vi "TestGenTabNameHeaders.vi"() -> ()   [LabVIEW 2014, in "TableLogger_Actor.lvlib" / "TableLogger_Actor.lvclass"]
uses:
  TableLogger_Actor.lvclass
  <userlib>/_OpenG.lib/lvdata/lvdata.llb/Type Descriptor Enumeration__ogtk.ctl
panel:
  out "LV Data Types 3":T1[](array[typedef]) format="%.0x"
  out "Headers 2":string[](array[string])
  out "Data 2":string[](array[string])
  out "LV Data Types 2":T1[](array[typedef]) format="%.0x"
  out "Table Name":string
  out "Headers":string[](array[string])
  out "Data":string[][](array[string])
  out "LV Data Types":T1[][](array[typedef]) format="%.0x"
  out "Table Names":string[](array[string])
  out "Column Headers":string[][](array[string])
  out "Column Data Types":string[][](array[string])
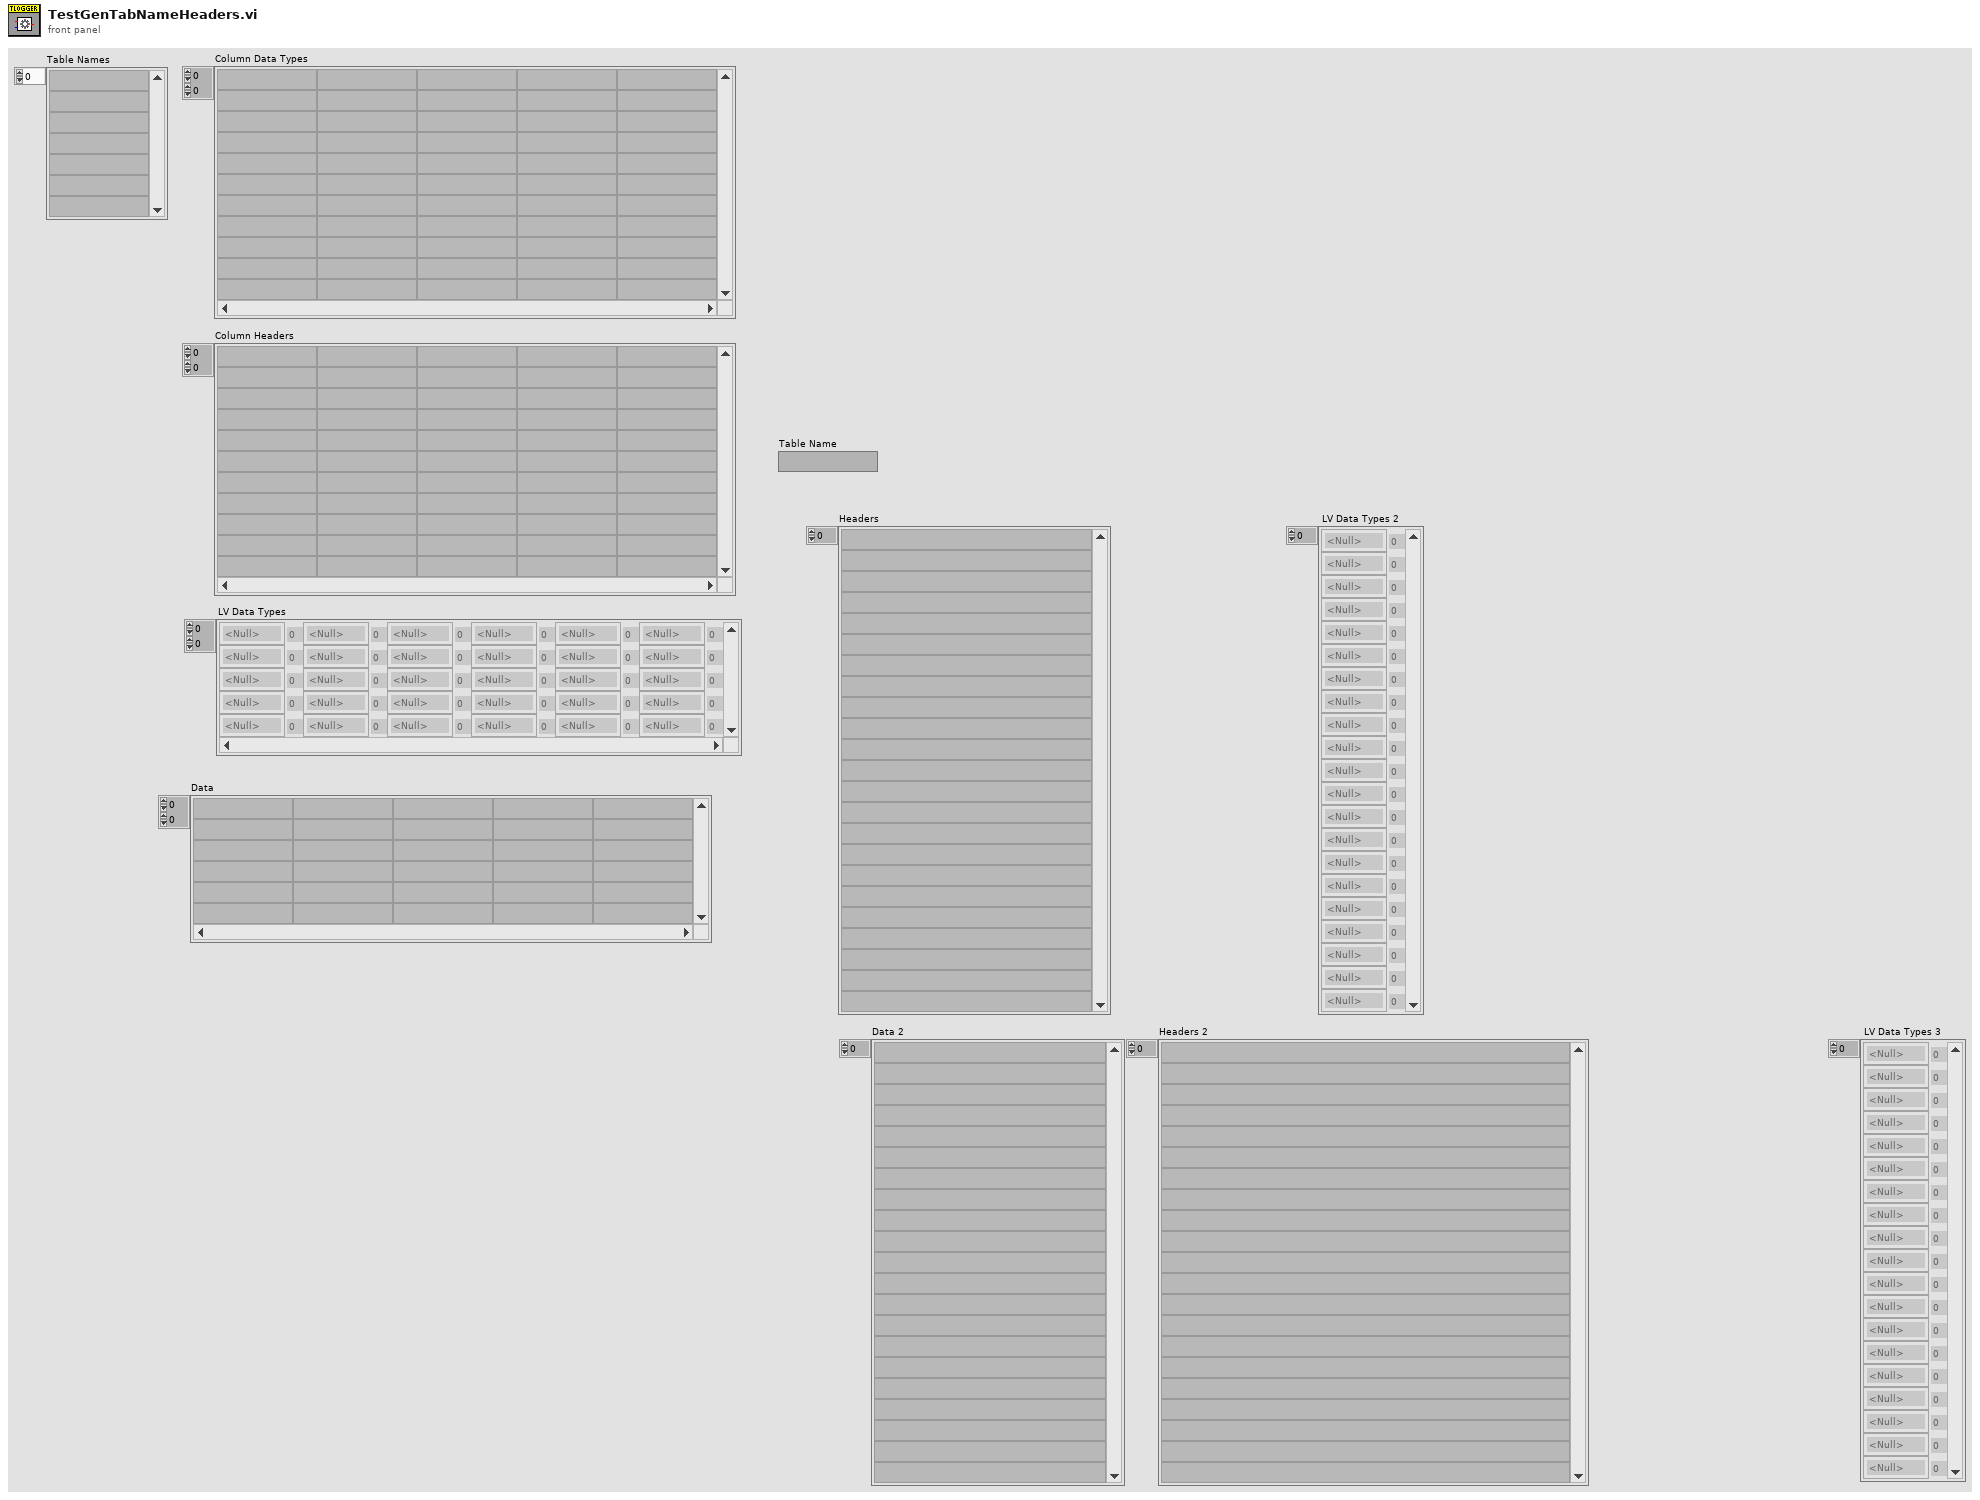
[diagram p1: front panel]
types:
  T1 = typedef "Type Descriptor Enumeration__ogtk.ctl" = enum8{"<Null>", "I8", "I16", "I32", "I64", "U8", "U16", "U32", "U64", "SGL", "DBL", "EXT", "CSG", "CDB", "CXT", "0x0F", "0x10", "0x11", "0x12", "0x13", "0x14", "Enum U8", "Enum U16", "Enum U32", "Enum U64", "SGL PQ", "DBL PQ", "EXT PQ", "CSG PQ", "CDB PQ", "CXT PQ", "0x1F", "0x20", "Boolean", "0x22", "0x23", "0x24", "0x25", "0x26", "0x27", "0x28", "0x29", "0x2A", "0x2B", "0x2C", "0x2D", "0x2E", "0x2F", "String", "0x31", "Path", "Pict", "0x34", "0x35", "0x36", "DAQ", "0x38", "0x39", "0x3A", "0x3B", "0x3C", "0x3D", "0x3E", "0x3F", "Array", "0x41", "0x42", "0x43", "0x44", "0x45", "0x46", "0x47", "0x48", "0x49", "0x4A", "0x4B", "0x4C", "0x4D", "0x4E", "0x4F", "Cluster", "0x51", "0x52", "Variant", "Waveform", "0x55", "0x56", "0x57", "0x58", "0x59", "0x5A", "0x5B", "0x5C", "0x5D", "0x5E", "0x5F", "0x60", "0x61", "0x62", "0x63", "0x64", "0x65", "0x66", "0x67", "0x68", "0x69", "0x6A", "0x6B", "0x6C", "0x6D", "0x6E", "0x6F", "Refnum"}
  T2 = cluster{"FC Flow Set":dbl, "FM Flow Measure":dbl, "UUT Data":dbl, "Stage 1  Flow Meas":cluster{"FC Flow Set":dbl, "FM Flow Measure":dbl, "UUT Data":dbl, "Dataset":cluster{"Site Number":i32, "Operator ID":string, "Calibration Result":enum16{"Pass", "Fail"}, "Stage 1  Flow Meas":cluster{"FC Flow Set":dbl, "FM Flow Measure":dbl, "UUT Data":dbl}[]}}[]}[]
  T3 = cluster{"Test Start Timestamp":timestamp, "Test End Timestamp":timestamp, "Test Jig Location":string, "Location Time Offset":string, "Test Jig ID":string, "Test Jig Fluid":enum16{"DI", "N2"}, "Test Jig Flow":enum16{"Low", "High"}, "Control Board SN":string, "Site Number":i32, "Operator ID":string, "Operation Number":string, "DUT Serial Number":string, "DUT Product Number":string, "DUT Flow Range":i32, "DUT FW Revision":string, "DUT TP1 Offset":dbl, "DUT TP2 Offset":dbl, "DUT Cut Off1":dbl, "DUT Cut Off2":dbl, "PreCal Flow Meas":cluster{"FC Flow Set":dbl, "FM Flow Measure":dbl, "UUT Data":dbl}[], "PostCal Flow Meas":cluster{"FC Flow Set":dbl, "FM Flow Measure":dbl, "UUT Data":dbl}[], "DUT_Coeff":dbl[], "DUT_Flow_Error":dbl[], "Calibration Result":enum16{"Pass", "Fail"}}
  T4 = cluster{"FC Flow Set":dbl, "FM Flow Measure":dbl, "UUT Data":dbl, "Stage 1  Flow Meas":cluster{"FC Flow Set":dbl, "FM Flow Measure":dbl, "UUT Data":dbl}[]}[]
  T5 = cluster{"Site Number":i32, "Operator ID":string, "Calibration Result":enum16{"Pass", "Fail"}, "Stage 1  Flow Meas":cluster{"FC Flow Set":dbl, "FM Flow Measure":dbl, "UUT Data":dbl}[]}
  T6 = cluster{"Site Number":i32, "Operator ID":string, "PreCal Flow Meas":cluster{"FC Flow Set":dbl, "FM Flow Measure":dbl, "UUT Data":dbl}[], "PostCal Flow Meas":cluster{"FC Flow Set":dbl, "FM Flow Measure":dbl, "UUT Data":dbl}[], "DUT_Coeff":dbl[], "DUT_Flow_Error":dbl[], "Calibration Result":enum16{"Pass", "Fail"}}
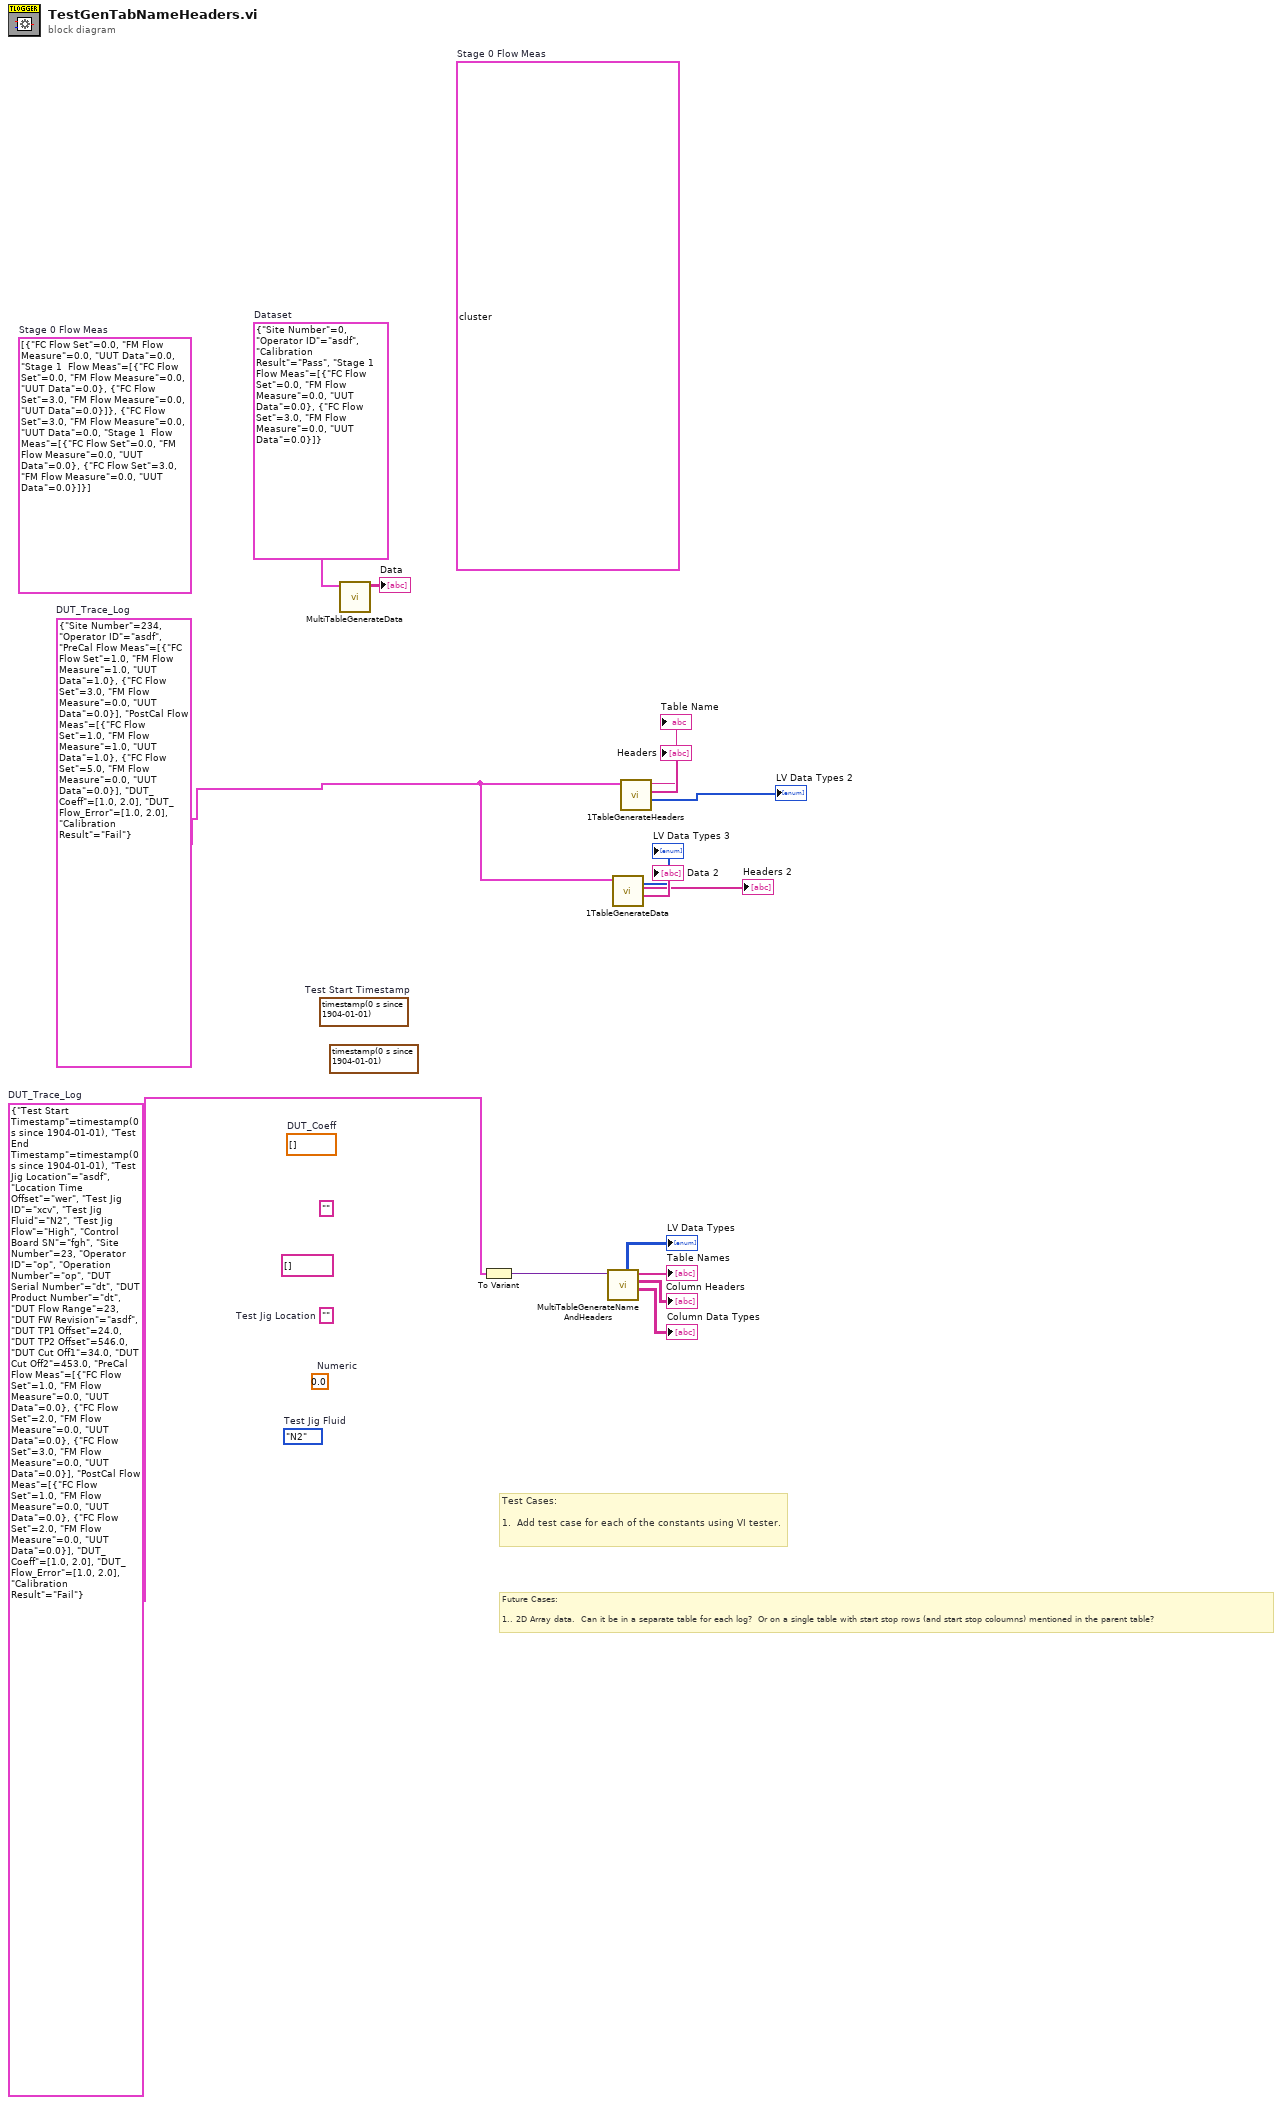
[diagram p0: block diagram]
diagram:
  (unwired) T2 [{"FC Flow Set"=0.0, "FM Flow Measure"=0.0, "UUT Data"=0.0, "Stage 1  Flow Meas"=[{"FC Flow Set"=0.0, "FM Flow Measure"=0.0, "UUT Data"=0.0, "Dataset"={"Site Number"=0, "Operator ID"="asdf", "Calibration Result"=enum."Pass", "Stage 1  Flow Meas"=[{"FC Flow Set"=0.0, "FM Flow Measure"=0.0, "UUT Data"=0.0}, {"FC Flow Set"=3.0, "FM Flow Measure"=0.0, "UUT Data"=0.0}]}}, {"FC Flow Set"=3.0, "FM Flow Measure"=0.0, "UUT Data"=0.0, "Dataset"={"Site Number"=0, "Operator ID"="asdf", "Calibration Result"=enum."Pass", "Stage 1  Flow Meas"=[{"FC Flow Set"=0.0, "FM Flow Measure"=0.0, "UUT Data"=0.0}, {"FC Flow Set"=3.0, "FM Flow Measure"=0.0, "UUT Data"=0.0}]}}]}, {"FC Flow Set"=3.0, "FM Flow Measure"=0.0, "UUT Data"=0.0, "Stage 1  Flow Meas"=[{"FC Flow Set"=0.0, "FM Flow Measure"=0.0, "UUT Data"=0.0, "Dataset"={"Site Number"=0, "Operator ID"="asdf", "Calibration Result"=enum."Pass", "Stage 1  Flow Meas"=[{"FC Flow Set"=0.0, "FM Flow Measure"=0.0, "UUT Data"=0.0}, {"FC Flow Set"=3.0, "FM Flow Measure"=0.0, "UUT Data"=0.0}]}}, {"FC Flow Set"=3.0, "FM Flow Measure"=0.0, "UUT Data"=0.0, "Dataset"={"Site Number"=0, "Operator ID"="asdf", "Calibration Result"=enum."Pass", "Stage 1  Flow Meas"=[{"FC Flow Set"=0.0, "FM Flow Measure"=0.0, "UUT Data"=0.0}, {"FC Flow Set"=3.0, "FM Flow Measure"=0.0, "UUT Data"=0.0}]}}]}]  # Stage 0 Flow Meas
  (unwired) enum16{"DI", "N2"}."N2"  # Test Jig Fluid
  (unwired) timestamp(0 s since 1904-01-01)  # Test Start Timestamp
  (unwired) timestamp(0 s since 1904-01-01)
  (unwired) ""
  (unwired) string[] []
  (unwired) ""  # Test Jig Location
  (unwired) 0.0  # Numeric
  (unwired) dbl[] []  # DUT_Coeff
  w4 = T3 {"Test Start Timestamp"=timestamp(0 s since 1904-01-01), "Test End Timestamp"=timestamp(0 s since 1904-01-01), "Test Jig Location"="asdf", "Location Time Offset"="wer", "Test Jig ID"="xcv", "Test Jig Fluid"=enum."N2", "Test Jig Flow"=enum."High", "Control Board SN"="fgh", "Site Number"=23, "Operator ID"="op", "Operation Number"="op", "DUT Serial Number"="dt", "DUT Product Number"="dt", "DUT Flow Range"=23, "DUT FW Revision"="asdf", "DUT TP1 Offset"=24.0, "DUT TP2 Offset"=546.0, "DUT Cut Off1"=34.0, "DUT Cut Off2"=453.0, "PreCal Flow Meas"=[{"FC Flow Set"=1.0, "FM Flow Measure"=0.0, "UUT Data"=0.0}, {"FC Flow Set"=2.0, "FM Flow Measure"=0.0, "UUT Data"=0.0}, {"FC Flow Set"=3.0, "FM Flow Measure"=0.0, "UUT Data"=0.0}], "PostCal Flow Meas"=[{"FC Flow Set"=1.0, "FM Flow Measure"=0.0, "UUT Data"=0.0}, {"FC Flow Set"=2.0, "FM Flow Measure"=0.0, "UUT Data"=0.0}], "DUT_Coeff"=[1.0, 2.0], "DUT_Flow_Error"=[1.0, 2.0], "Calibration Result"=enum."Fail"}  # DUT_Trace_Log
  (unwired) T4 [{"FC Flow Set"=0.0, "FM Flow Measure"=0.0, "UUT Data"=0.0, "Stage 1  Flow Meas"=[{"FC Flow Set"=0.0, "FM Flow Measure"=0.0, "UUT Data"=0.0}, {"FC Flow Set"=3.0, "FM Flow Measure"=0.0, "UUT Data"=0.0}]}, {"FC Flow Set"=3.0, "FM Flow Measure"=0.0, "UUT Data"=0.0, "Stage 1  Flow Meas"=[{"FC Flow Set"=0.0, "FM Flow Measure"=0.0, "UUT Data"=0.0}, {"FC Flow Set"=3.0, "FM Flow Measure"=0.0, "UUT Data"=0.0}]}]  # Stage 0 Flow Meas
  w2 = T5 {"Site Number"=0, "Operator ID"="asdf", "Calibration Result"=enum."Pass", "Stage 1  Flow Meas"=[{"FC Flow Set"=0.0, "FM Flow Measure"=0.0, "UUT Data"=0.0}, {"FC Flow Set"=3.0, "FM Flow Measure"=0.0, "UUT Data"=0.0}]}  # Dataset
  w1 = T6 {"Site Number"=234, "Operator ID"="asdf", "PreCal Flow Meas"=[{"FC Flow Set"=1.0, "FM Flow Measure"=1.0, "UUT Data"=1.0}, {"FC Flow Set"=3.0, "FM Flow Measure"=0.0, "UUT Data"=0.0}], "PostCal Flow Meas"=[{"FC Flow Set"=1.0, "FM Flow Measure"=1.0, "UUT Data"=1.0}, {"FC Flow Set"=5.0, "FM Flow Measure"=0.0, "UUT Data"=0.0}], "DUT_Coeff"=[1.0, 2.0], "DUT_Flow_Error"=[1.0, 2.0], "Calibration Result"=enum."Fail"}  # DUT_Trace_Log
  # "Test Cases:\n\n1.  Add test case for each of the constants using VI tester."
  # "Future Cases: \n\n1.. 2D Array data.  Can it be in a separate table for each log?  Or on a single table with start stop rows (and start stop coloumns) mentioned in the parent table?"
  n1 = call "MultiTableGenerateData.vi"("Cluster Variant"=w2) -> ("Data"=→"Data":string[][])  [unwired: 9 in, 1 out]
  n2 = To Variant(anything=w4) -> (Variant=w15:variant)
  n3 = call "MultiTableGenerateNameAndHeaders.vi"("Cluster Variant"=w15) -> ("SQL Data Types"=→"Column Data Types":string[][], "Headers"=→"Column Headers":string[][], "Table Names"=→"Table Names":string[], "LV Data Types"=→"LV Data Types":T1[][])  [unwired: 6 in, 1 out]
  n4 = call "1TableGenerateData.vi"("Cluster Variant"=w1) -> ("Data"=→"Data 2":string[], "Headers"=→"Headers 2":string[], "LV Data Types"=→"LV Data Types 3":T1[])  [unwired: 6 in, 2 out]
  n5 = call "1TableGenerateHeaders.vi"("Cluster Variant"=w1) -> ("LV Data Types"=→"LV Data Types 2":T1[], "Headers"=→"Headers":string[], "Table Name"=→"Table Name":string)  [unwired: 7 in, 1 out]
